vi "2.4.vi"() -> ()   [LabVIEW 2017]
uses:
  sin.vi
panel:
  in  "簇":cluster{"学生学号":i32, "学生姓名":string, "注册情况":bool} {"学生学号" step=1}
  out "是否注册":bool
  out "学号":i32
  out "姓名":string
  in  "停止":bool
  # "任务四"
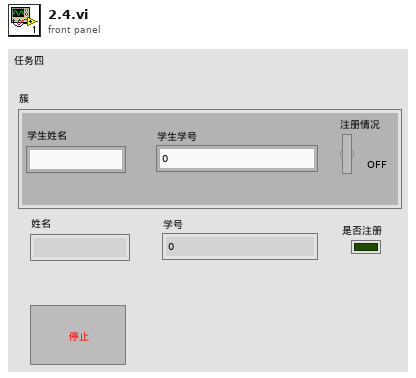
[diagram p1: front panel]
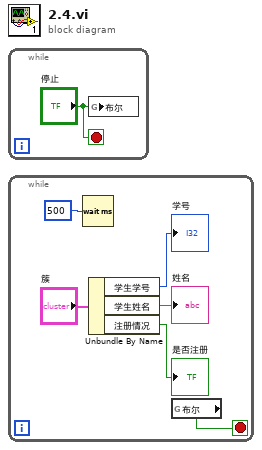
[diagram p0: block diagram]
diagram:
  n1 = while {
    stop <- "停止" stop-if-true
    n2 = global write "sin.vi" "布尔"("停止") -> ()
  }
  n3 = while {
    stop <- w7 stop-if-true
    n4 = Wait (ms)(milliseconds to wait=500) -> ()  [unwired: 1 out]
    n5 = Unbundle By Name("簇") -> ("学生学号"=→"学号":i32, "学生姓名"=→"姓名":string, "注册情况"=→"是否注册":bool)
    n6 = global read "sin.vi" "布尔"() -> (w7:bool)
  }
